vi "FilePaths.vi"(8 "error in":errorcluster) -> (0 "error out":errorcluster, 2 "paths":T1)   [LabVIEW 2015, in "Configuration Tool.lvlib"]
doc: "This VI has the Path to the Classes and the Glyphs, Additional Behavior might be added if you want to load them from a different path. By default they are in Glyphs folder and Classes folder in the main directoryCopyright 2017 National Instruments Corporation\n\nLicensed under the Apache License, Version 2.0 (the \"License\"); you may not use this file except in compliance with the License. You may obtain a copy of the License at http://www.apache.org/licenses/LICENSE-2.0\nUnless required by applicable law or agreed to in writing, software distributed under the License is distributed on an \"AS IS\" BASIS, WITHOUT WARRANTIES OR CONDITIONS OF ANY KIND, either express or implied. See the License for the specific language governing permissions and limitations under the License."
uses:
  Configuration Tool.lvlib
  Controls/FilePaths.ctl
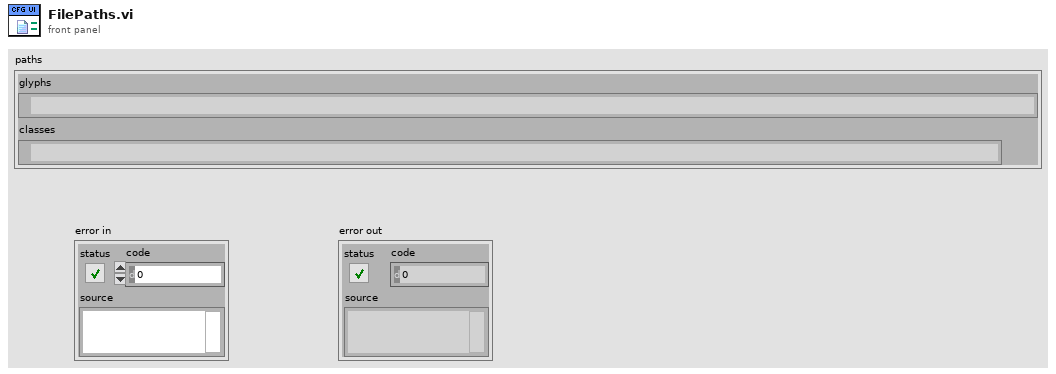
[diagram p1: front panel]
types:
  T1 = typedef "Configuration Tool.lvlib/FilePaths.ctl" = cluster{"glyphs":path, "classes":path}
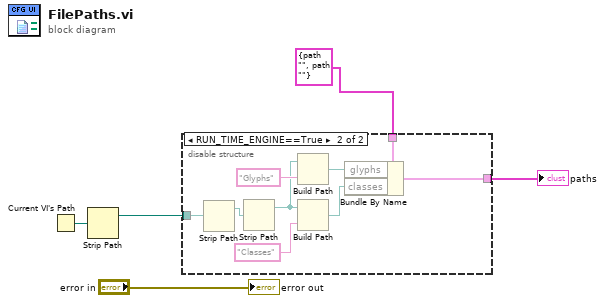
[diagram p0: block diagram]
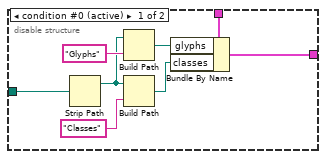
[diagram p2: hidden frame]
diagram:
  n1 = Current VI's Path() -> (path=w2:path)
  n2 = Strip Path(path=w2) -> (stripped path=w1:path)  [unwired: 1 out]
  n3 = disable-structure shown="RUN_TIME_ENGINE==True" {
    disable-tunnel: T1 {"glyphs"=path "", "classes"=path ""} ("Cluster 2") -> [w13 w22]
    disable-tunnel: [w12 w21] -> w4
    disable-tunnel: w1 -> [w8 w15]
    frame condition #0 (active) {
      n4 = Strip Path(path=w8) -> (stripped path=w9:path)  [unwired: 1 out]
      n5 = Build Path(base path=w9, name or relative path="Glyphs") -> (appended path=w6:path)
      n6 = Build Path(base path=w9, name or relative path="Classes") -> (appended path=w7:path)
      n7 = Bundle By Name(cluster=w13, "glyphs"=w6, "classes"=w7) -> (w12:T1)
    }
    frame condition #1 {
      n8 = Strip Path(path=w15) -> (stripped path=w14:path)  [unwired: 1 out]
      n9 = Strip Path(path=w14) -> (stripped path=w18:path)  [unwired: 1 out]
      n10 = Build Path(base path=w18, name or relative path="Glyphs") -> (appended path=w16:path)
      n11 = Build Path(base path=w18, name or relative path="Classes") -> (appended path=w17:path)
      n12 = Bundle By Name(cluster=w22, "glyphs"=w16, "classes"=w17) -> (w21:T1)
    }
  }
  "paths" <- w4
  "error out" <- "error in"
